vi "Get Credentials.vi"(8 "error in":errorcluster, 11 "IP Address":string) -> (0 "error out":errorcluster, 2 "Password":string, 3 "User name":string)   [LabVIEW 2020]
doc: "This VI pops up into the screen to get the device credentials."
panel:
  in  "OK Button":bool
  in  "Password":string
  in  "User name":string
  out "Message":string
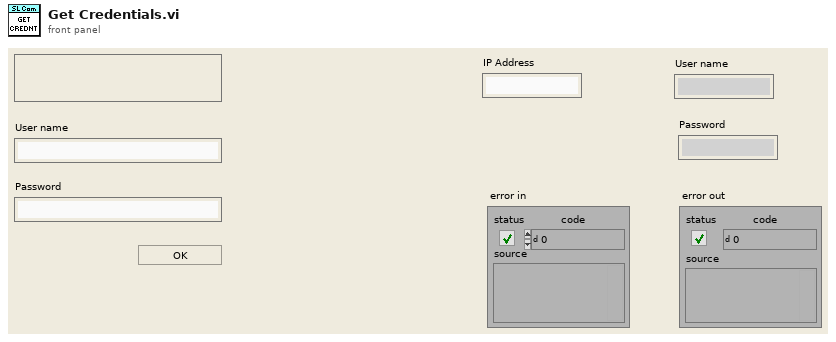
[diagram p1: front panel]
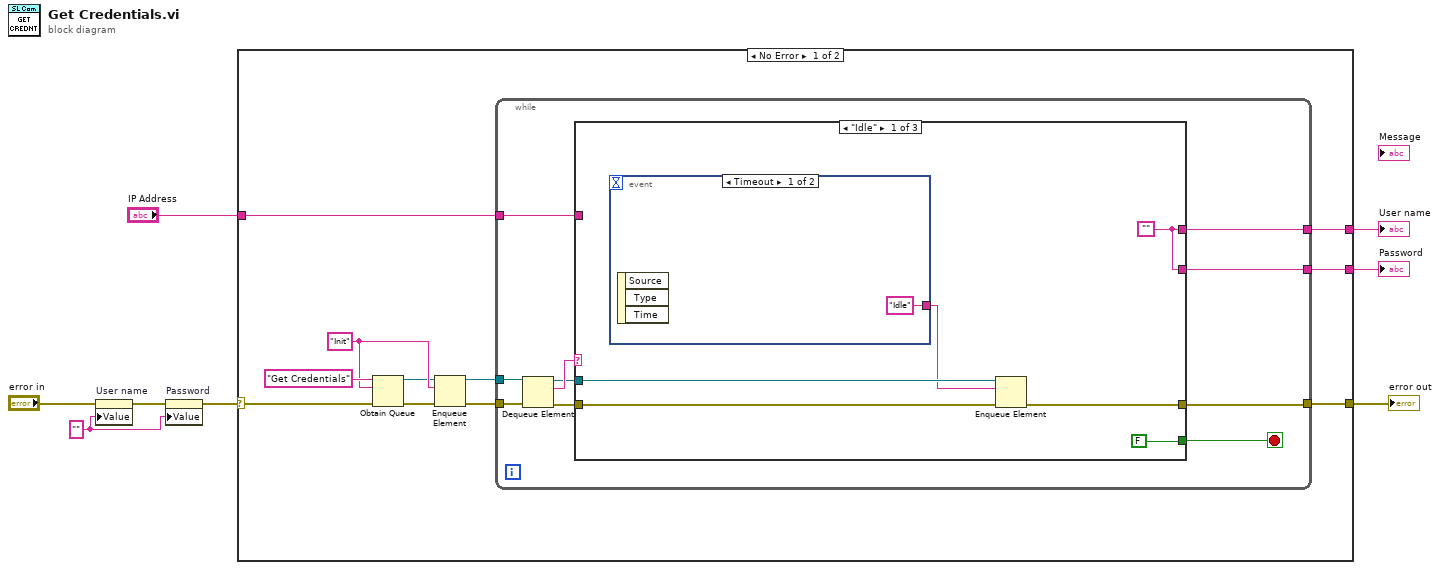
[diagram p0: block diagram]
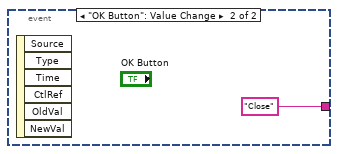
[diagram p2: hidden frame]
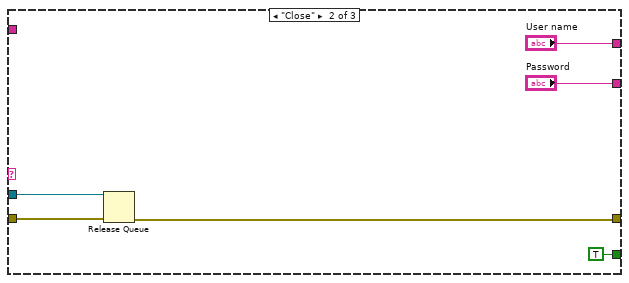
[diagram p3: hidden frame]
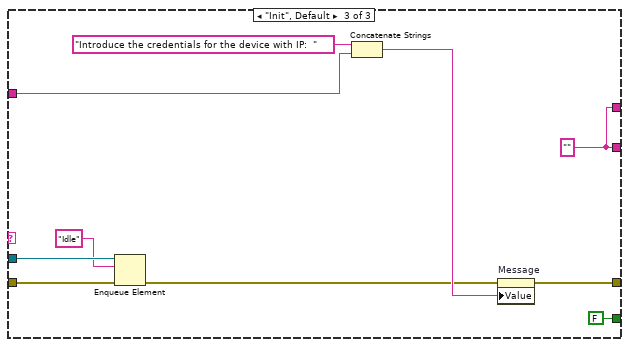
[diagram p4: hidden frame]
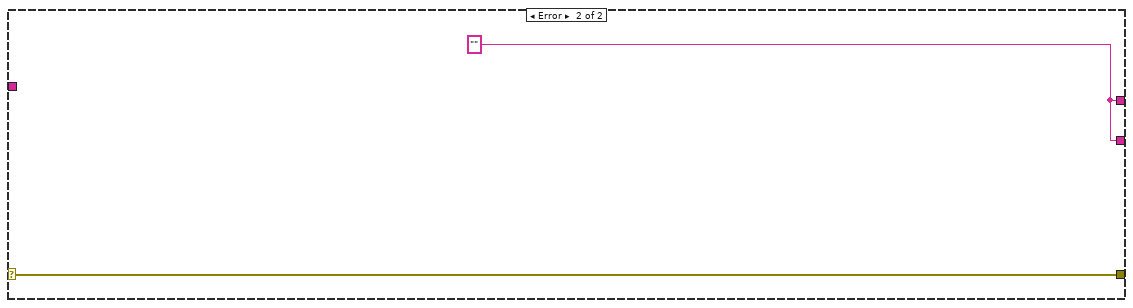
[diagram p5: hidden frame]
diagram:
  w1 = "" ("Password")
  n1 = property on="User name" class="Str"(error in="error in", "Value"=w1) -> (error out=w3:errorcluster)  [unwired: 1 in, 1 out]
  n2 = property on="Password" class="Str"(error in=w3, "Value"=w1) -> (error out=w4:errorcluster)  [unwired: 1 in, 1 out]
  n3 = case shown="No Error" w4 {
    selector: w4 -> [w11 w55]
    tunnel: "IP Address" -> [w19 _]
    tunnel: [w18 w54] -> w7
    tunnel: [w17 w54] -> w6
    tunnel: [w16 w55] -> w5
    frame No Error {
      w14 = "Init" ("name (unnamed)")
      n4 = Obtain Queue(name (unnamed)="Get Credentials", element data type=w14, error in (no error)=w11) -> (queue out=w13:refnum<queue>, error out=w12:errorcluster)  [unwired: 2 in, 1 out]
      n5 = Enqueue Element(queue=w13, element=w14, error in (no error)=w12) -> (queue out=w9:refnum<queue>, error out=w10:errorcluster)  [unwired: 1 in, 1 out]
      n6 = while {
        tunnel: [w22] -> w18
        tunnel: [w21] -> w17
        tunnel: [w25] -> w16
        tunnel: w19 -> [w26]
        tunnel: w10 -> [w29]
        tunnel: w9 -> [w24]
        stop <- w20 stop-if-true
        n7 = Dequeue Element(queue=w24, error in (no error)=w29) -> (queue out=w23:refnum<queue>, element=w28:string, error out=w27:errorcluster)  [unwired: 1 in, 1 out]
        n8 = case shown="\"Idle\"" w28 {
          tunnel: w27 -> [w35 w42 w49]
          tunnel: w26 -> [_ _ w52]
          tunnel: [w32 w41 w50] -> w25
          tunnel: w23 -> [w34 w43 w48]
          tunnel: [w30 "User name" w45] -> w22
          tunnel: [w30 "Password" w45] -> w21
          tunnel: [FALSE TRUE FALSE] -> w20
          frame "Idle" {
            w30 = "" ("element")
            n9 = event shown="[0] Timeout" {
              selector: _ -> [_ _]
              dyn-events: _ -> [_ _]
              timeout: _ -> [_ _]
              tunnel: ["Idle" ("element") "Close" ("element")] -> w33
              event Timeout {
                n10 = event-data() -> ()  [unwired: 1 in, 3 out]
              }
              event "OK Button": Value Change {
                n11 = event-data() -> ()  [unwired: 1 in, 6 out]
              }
            }
            n12 = Enqueue Element(queue=w34, element=w33, error in (no error)=w35) -> (error out=w32:errorcluster)  [unwired: 1 in, 2 out]
          }
          frame "Close" {
            n13 = Release Queue(queue=w43, error in (no error)=w42) -> (error out=w41:errorcluster)  [unwired: 1 in, 2 out]
          }
          frame "Init", Default {
            w45 = "" ("element")
            n14 = Enqueue Element(queue=w48, element="Idle", error in (no error)=w49) -> (error out=w46:errorcluster)  [unwired: 1 in, 2 out]
            n15 = Concatenate Strings("Introduce the credentials for the device with IP:  " ("string"), w52) -> (w51:string)
            n16 = property on="Message" class="Str"(error in=w46, "Value"=w51) -> (error out=w50:errorcluster)  [unwired: 1 in, 1 out]
          }
        }
      }
    }
    frame Error {
      w54 = ""
    }
  }
  "User name" <- w7
  "Password" <- w6
  "error out" <- w5
